vi "Alpha start.vi"() -> ()   [LabVIEW 2019]
doc: "Thus VI communicates with \"omega\" via the collection of global variables in \"tau\".\n\nIf stopped, it stops \"omega\" as well automatically.\n\nJuan Gamez\nP3600\nCSUSB Physics"
uses:
  globals/Tau start.vi
panel:
  out "Active":bool
  in  "publish info":bool
  out "text read from global":string
  out "number read from global":dbl
  in  "text to publish":string="Hello Omega"
  in  "number to publish":dbl=3.0
  in  "grab info":bool
  in  "stop both":bool
  # "Juan Gamez\np3600"
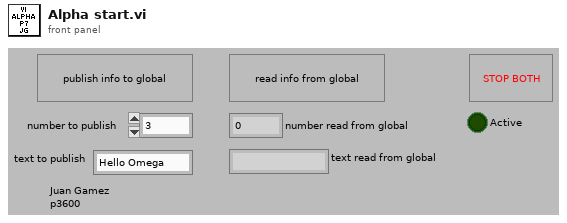
[diagram p1: front panel]
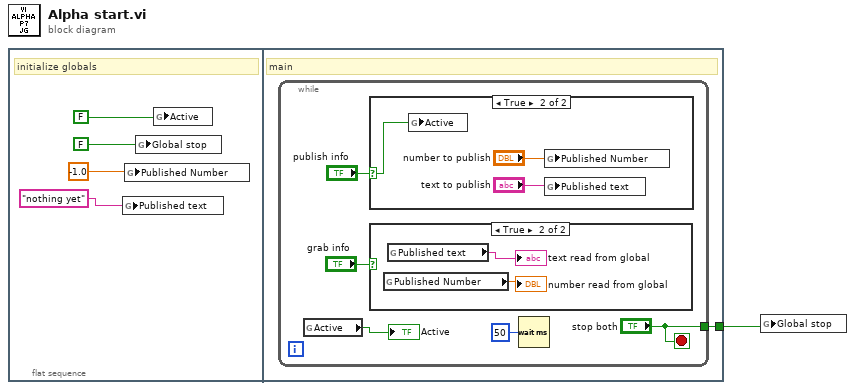
[diagram p0: block diagram]
diagram:
  n1 = flat-sequence {
    tunnel: [w6] -> w1
    frame #0 {
      # "initialize globals"
      n2 = global write "Tau start.vi" "Published text"("nothing yet" ("published text")) -> ()
      n3 = global write "Tau start.vi" "Published Number"(-1.0 ("published number")) -> ()
      n4 = global write "Tau start.vi" "Global stop"(FALSE ("global stop")) -> ()
      n5 = global write "Tau start.vi" "Active"(FALSE ("Active")) -> ()
    }
    frame #1 {
      # "main"
      n6 = while {
        tunnel: ["stop both"] -> w6
        stop <- "stop both" stop-if-true
        n7 = global read "Tau start.vi" "Active"() -> (→"Active":bool)
        n8 = case shown="True" "publish info" {
          selector: "publish info" -> [_ w14]
          frame False {
          }
          frame True {
            n9 = global write "Tau start.vi" "Active"(w14) -> ()
            n10 = global write "Tau start.vi" "Published Number"("number to publish") -> ()
            n11 = global write "Tau start.vi" "Published text"("text to publish") -> ()
          }
        }
        n12 = case shown="True" "grab info" {
          frame False {
          }
          frame True {
            n13 = global read "Tau start.vi" "Published Number"() -> (→"number read from global":dbl)
            n14 = global read "Tau start.vi" "Published text"() -> (→"text read from global":string)
          }
        }
        n15 = Wait (ms)(milliseconds to wait=u32 50) -> ()  [unwired: 1 out]
      }
    }
  }
  n16 = global write "Tau start.vi" "Global stop"(w1) -> ()
